vi "MemoryStateValid.vi"() -> ()   [LabVIEW 2020, in "Active Technologies AWG3000.lvlib"]
uses:
  Active Technologies AWG3000.lvlib
panel:
  in  "Configuration Name":string
  out "Memory State":u8(ring) items=["Available", "Occupied"]
  in  "Select Setup Memory / Configuration":u16(ring) items=["Memory 0", "Memory 1", "Memory 2", "Memory 3", "Memory 4", "Configuration"]
  in  "error in (no error)":errorcluster
  out "error out":errorcluster
  out "VISA resource name out":refnum<visa-resource-name>
  in  "VISA resource name":refnum<visa-resource-name>
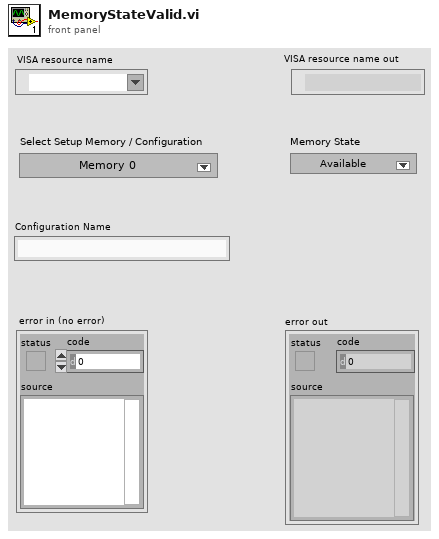
[diagram p1: front panel]
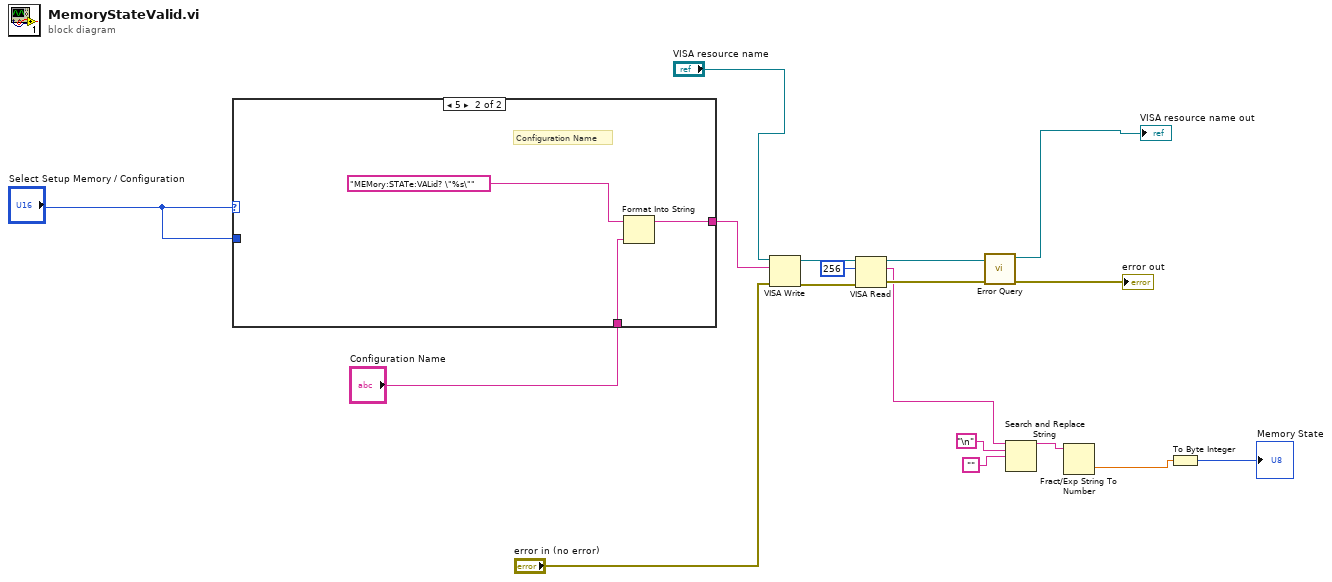
[diagram p0: block diagram]
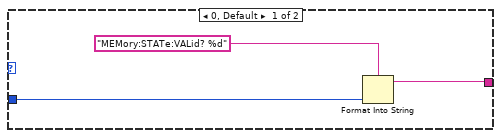
[diagram p2: hidden frame]
diagram:
  n1 = case shown="5" "Select Setup Memory / Configuration" {
    tunnel: [w20 w23] -> w13
    tunnel: "Configuration Name" -> [_ w22]
    tunnel: "Select Setup Memory / Configuration" -> [w19 _]
    frame 0, Default {
      n2 = Format Into String(format string="MEMory:STATe:VALid? %d" ("write buffer"), w19) -> (resulting string=w20:string)  [unwired: 2 in, 1 out]
    }
    frame 5 {
      # "Configuration Name"
      n3 = Format Into String(format string="MEMory:STATe:VALid? \"%s\"" ("write buffer"), w22) -> (resulting string=w23:string)  [unwired: 2 in, 1 out]
    }
  }
  n4 = VISA Write(VISA resource name="VISA resource name", write buffer=w13, error in (no error)="error in (no error)") -> (VISA resource name out=w18:refnum<visa-resource-name>, error out=w17:errorcluster)  [unwired: 1 out]
  n5 = VISA Read(VISA resource name=w18, byte count=u32 256, error in (no error)=w17) -> (VISA resource name out=w15:refnum<visa-resource-name>, read buffer=w8:string, error out=w14:errorcluster)  [unwired: 1 out]
  n6 = call "Error Query.vi"("error in (no error)"=w14, "VISA resource name"=w15) -> ("error out"=→"error out":errorcluster, "VISA resource name out"=→"VISA resource name out":refnum<visa-resource-name>)  [unwired: 6 in, 2 out]
  n7 = Search and Replace String(input string=w8, search string="\n", replace string="") -> (result string=w11:string)  [unwired: 5 in, 3 out]
  n8 = Fract/Exp String To Number(string=w11) -> (number=w10:dbl)  [unwired: 3 in, 1 out]
  n9 = To Byte Integer(number=w10) -> (8bit integer=→"Memory State":i8)
